vi "Motor_Simulation.vi"(6 "Cluster":cluster{"b":dbl, "a2":dbl, "a1":dbl, "a0":dbl}, 8 "Position":dbl, 9 "Velocity":dbl, 10 "Input (Vm)":dbl, 11 "dt":dbl) -> (0 "Position":dbl, 1 "Velocity":dbl)   [LabVIEW 2017]
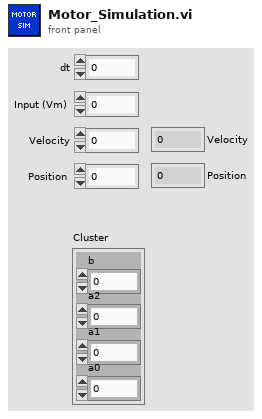
[diagram p1: front panel]
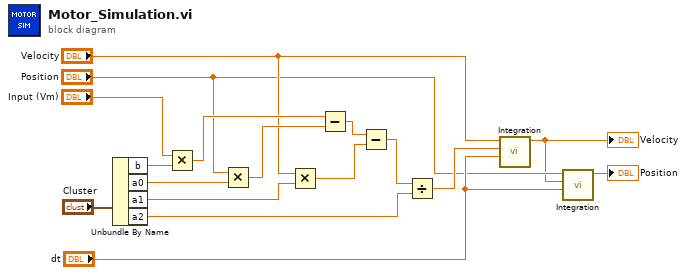
[diagram p0: block diagram]
diagram:
  n1 = Unbundle By Name("Cluster") -> ("b"=w12:dbl, "a0"=w16:dbl, "a1"=w15:dbl, "a2"=w14:dbl)
  n2 = Multiply(x="Input (Vm)", y=w12) -> (x*y=w11:dbl)
  n3 = Multiply(x="Position", y=w16) -> (x*y=w9:dbl)
  n4 = Multiply(x="Velocity", y=w15) -> (x*y=w8:dbl)
  n5 = Subtract(x=w11, y=w9) -> (x-y=w10:dbl)
  n6 = Subtract(x=w10, y=w8) -> (x-y=w7:dbl)
  n7 = Divide(x=w7, y=w14) -> (x/y=w6:dbl)
  n8 = call "Integration.vi"("dt"="dt", "x_dot"=w6, "x(n-1)"="Velocity") -> ("x(n)"=w1:dbl)  [unwired: 8 in]
  "Velocity" <- w1
  n9 = call "Integration.vi"("dt"="dt", "x_dot"=w1, "x(n-1)"="Position") -> ("x(n)"=→"Position":dbl)  [unwired: 8 in]
